vi "XNET Write (Signal Waveform) .vi"(0 "session in":refnum<k21>, 5 "data":waveform(dbl)[](array[waveform]), 9 "timeout (10)":dbl=10.0 format="%.2g", 11 "error in (no error)":errorcluster) -> (4 "session out":refnum<k21>, 15 "error out":errorcluster)   [LabVIEW 2018]
doc: "Writes data to a session of Signal Output Waveform mode. The data represents a waveform of resampled values for each signal in the session."
uses:
  nixlvapi.dll
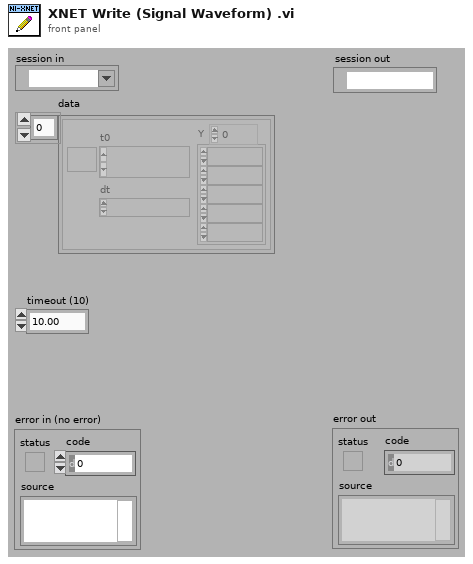
[diagram p1: front panel]
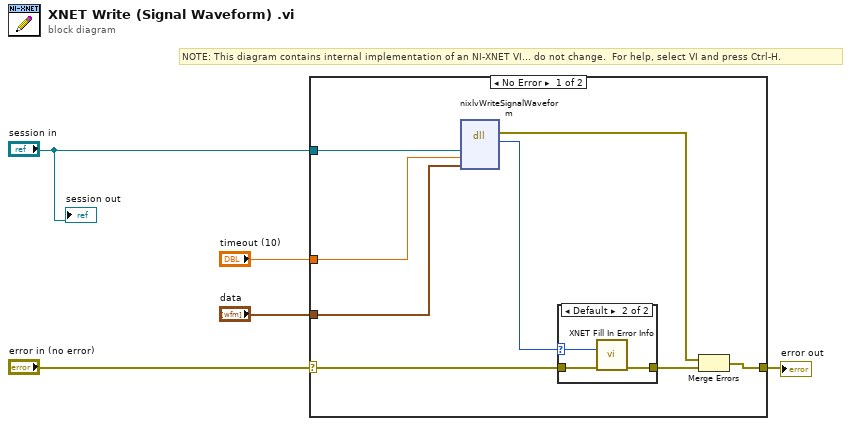
[diagram p0: block diagram]
diagram:
  # "NOTE: This diagram contains internal implementation of an NI-XNET VI... do not change.  For help, select VI and press Ctrl-H."
  n1 = case shown="No Error" "error in (no error)" {
    selector: "error in (no error)" -> [w12 w18]
    tunnel: "session in" -> [w11 _]
    tunnel: [w7 w18] -> w5
    tunnel: "data" -> [w8 _]
    tunnel: "timeout (10)" -> [w9 _]
    frame No Error {
      n2 = dll-call lib="nixlvapi.*" fn="nixlvWriteSignalWaveform"("SessionRef"=w11, "Timeout"=w9, "Data"=w8) -> (error out=w6:errorcluster, "return type"=w10:i32)  [unwired: 5 in, 2 out]
      n3 = case shown="Default" w10 {
        selector: w10 -> [_ w15]
        tunnel: w12 -> [w14 w16]
        tunnel: [w14 w17] -> w13
        frame 0 {
        }
        frame Default {
          n4 = call "XNET Fill In Error Info.vi"("status code"=w15, "error in"=w16) -> ("error out"=w17:errorcluster)  [unwired: 13 out]
        }
      }
      n5 = Merge Errors(w6, w13) -> (w7:errorcluster)
    }
    frame Error {
    }
  }
  "error out" <- w5
  "session out" <- "session in"
